vi "CF-recording_filepath.vi"(11 "Input path":string) -> (2 "data Path + input":path, 3 "data Path":path)   [LabVIEW 2020, in "CF-common_features.lvlib"]
uses:
  CF-common_features.lvlib
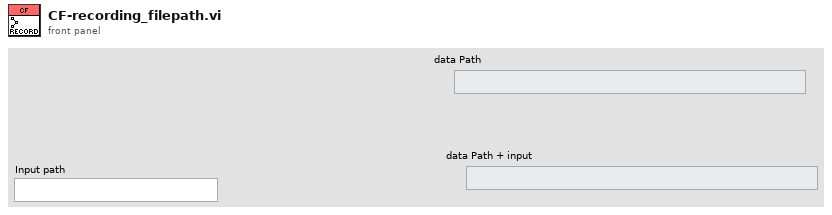
[diagram p1: front panel]
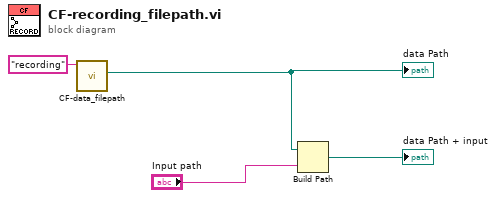
[diagram p0: block diagram]
diagram:
  n1 = call "CF-data_filepath.vi"("Input path"="recording") -> ("data Path + input"=w1:path)  [unwired: 9 in, 1 out]
  "data Path" <- w1
  n2 = Build Path(base path=w1, name or relative path="Input path") -> (appended path=→"data Path + input":path)
